vi "TEST_L1_COMPLETE_V2.vi"() -> ()   [LabVIEW 2012]
uses:
  <vilib>/Utility/NIReport.llb/NI_report.lvclass
  <vilib>/Utility/NIReport.llb/HTML/NI_HTML.lvclass
  Sum_Abrilader/L0_Sum_Adder Folder/C/Program Files/National Instruments/LabVIEW 2012/instr.lib/Agilent 8000 Series/Public/Data/Low Level/Fetch Measurement (More).vi
  <instrlib>/Agilent 8000 Series/Agilent 8000 Series.lvlib
  Sum_Abrilader/L0_Sum_Adder Folder/C/Program Files/National Instruments/LabVIEW 2012/instr.lib/Agilent 81150/Agilent 81150.lvlib
panel:
  in  "Default register":u16[](array[numeric])=[2389, 32764, 32767, 32767, 16384, 160, 6656]
  out "Current Channel":i32
  in  "Pulse Amplitudes":dbl[](array[numeric])=[0.3]
  out "IPR_count":u32=1000
  in  "step":i32=10
  in  "min DT":i32
  in  "max DT":dbl=200.0
  in  "Gains":dbl[](array[numeric])=[0.96, 0.97, 0.98, 0.88, 1.0, 1.0, 0.99]
  in  "Instrument VISA in":T1={"AWG VISA"="AgilentGenerator1", "Oscilloscope  VISA "="AgilentOsciloscope", "Integration Board IP"="172.16.17.48", "connection ID"=refnum, "report out"=refnum, "report file path"=path "C:/Users/omartinez/Desktop/L0nL1_Results"}
  out "data out serial":string="empty_read_bufferwrittingempty_read_bufferwritting2"
  in  "Combination\n  (Act High)":i32 min=0 max=127 step=1 format="%b"
  in  "Single/Comb":bool=TRUE
  in  "Single Channel Enable":i32(slide) scale=0.0..6.0
  out "error out":errorcluster
  in  "error in":errorcluster
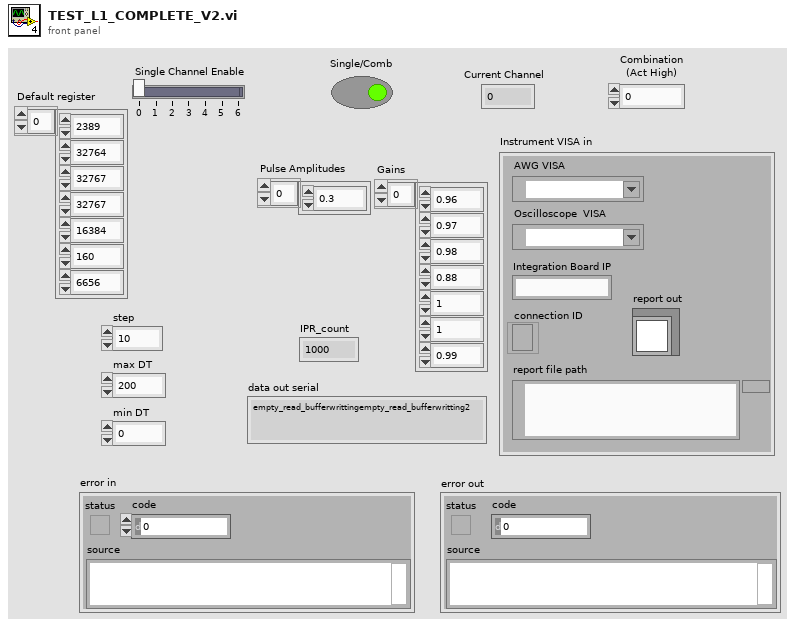
[diagram p1: front panel]
types:
  T1 = cluster{"AWG VISA":refnum<visa-resource-name>, "Oscilloscope  VISA ":refnum<visa-resource-name>, "Integration Board IP":string, "connection ID":refnum<k5>, "report out":refnum<class "NI_report.lvclass">, "report file path":path}
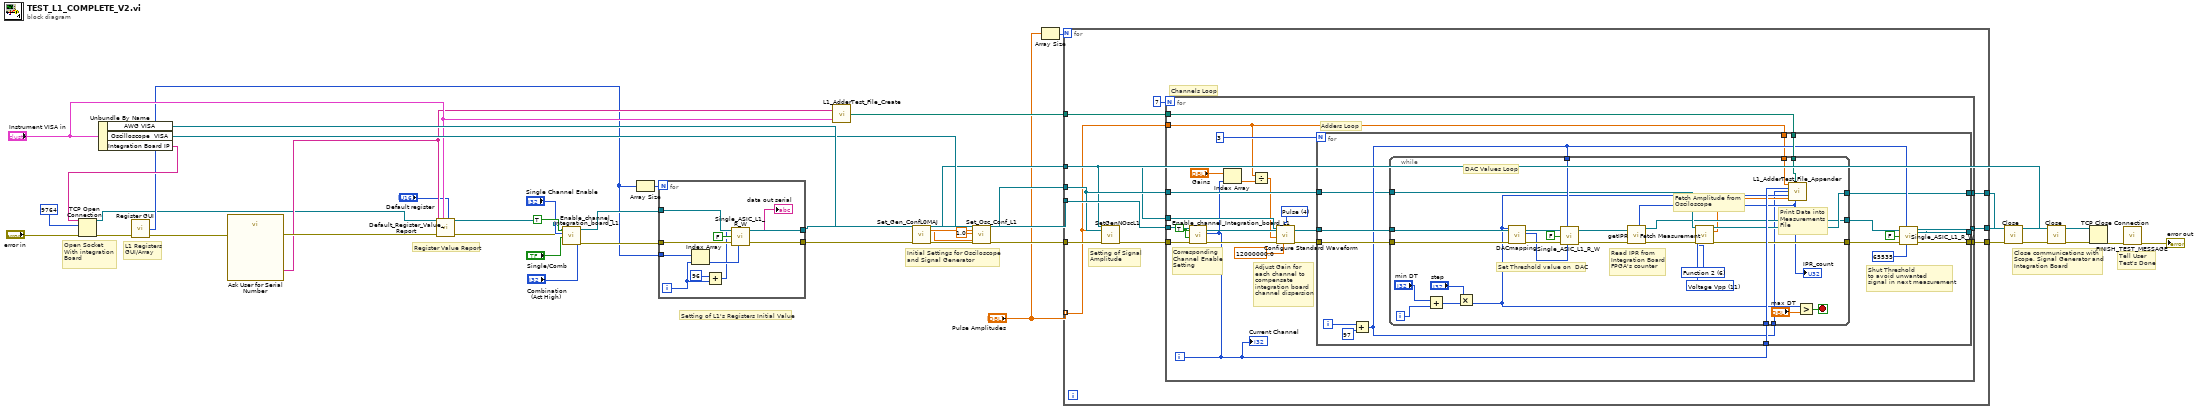
[diagram p0: block diagram]
diagram:
  # "Register Value Report"
  # "Tell User\nTest's Done"
  # "Close communications with \nScope, Signal Generator and \nIntegration Board"
  # "Initial Settings for Osciloscope\nand Signal Generator"
  # "Setting of L1's Registers Initial Value"
  # "L1 Registers\nGUI/Array"
  # "Open Socket\nWith integration \nBoard"
  n1 = Unbundle By Name("Instrument VISA in") -> ("AWG VISA"=w25:refnum<visa-resource-name>, "Oscilloscope  VISA"=w24:refnum<visa-resource-name>, "Integration Board IP"=w31:string)
  n2 = TCP Open Connection(address=w31, remote port or service name=9764, error in (no error)="error in") -> (connection ID=w3:refnum<k5>, error out=w12:errorcluster)  [unwired: 2 in]
  n3 = call "Register GUI.vi"("error in (no error)"=w12) -> ("error out"=w11:errorcluster, "REG ARRAy"=w4:u32[])  [unwired: 3 in]
  n4 = call "Ask User for Serial Number"("error in (no error)"=w11) -> ("Serial Number"=w5:string, "error out"=w7:errorcluster)  [unwired: 16 in, 1 out]
  n5 = call "Default_Register_Value_Report.vi"("Default register"="Default register", "input cluster"="Instrument VISA in", "error out"=w7, "Serial Number"=w5, "connection ID"=w3) -> ("error out 2"=w8:errorcluster, "connection ID out"=w2:refnum<k5>)  [unwired: 4 in, 1 out]
  n6 = call "Enable_channel_Integration_board_L1.vi"("Cobination"="Combination\n  (Act High)", "Enable  L1 single  Input"="Single Channel Enable", "error in (no error)"=w8, "SingleIN/#Combination"="Single/Comb", "#Enable all L1"=TRUE, "connection ID"=w2) -> ("error out"=w9:errorcluster, "connection ID out"=w33:refnum<k5>)
  n7 = Array Size(array=w4) -> (size(s)=w34:i32)
  n8 = for {
    N: w34 -> [_]
    tunnel: w9 -> [w52]
    tunnel: w4 -> [w51]
    tunnel: w33 -> [w50]
    tunnel: [w49] -> w29
    tunnel: [w48] -> w10
    i -> [w43]
    n9 = Index Array(array=w51, index=w43) -> (element=w47:u32)
    n10 = Add(x=96 ("y"), y=w43) -> (x+y=w45:i32)
    n11 = call "Single_ASIC_L1_R_W.vi"("connection ID"=w50, "Register or channel"=w45, "RD/#WR"=FALSE, "error in (no error)"=w52, "Data"=w47) -> ("data out serial"=→"data out serial":string, "connection ID out"=w49:refnum<k5>, "error out"=w48:errorcluster)  [unwired: 1 in, 1 out]
  }
  n12 = call "L1_AdderTest_File_Create.vi"("input cluster"="Instrument VISA in", "Serial Number"=w5) -> ("appended path"=w30:path)
  n13 = call "Set_Gen_ConfL0MAJ.vi"("AWG VISA"=w25, "error in (no error)"=w10) -> ("Amplitude 1 OUT"=w27:dbl, "VISA resource name out"=w16:refnum<visa-resource-name>, "Pulse Width in seconds 1 OUT"=w26:dbl, "error out"=w28:errorcluster)  [unwired: 10 in, 4 out]
  n14 = call "Set_Osc_Conf_L1.vi"("VISA resource name"=w24, "Amplitude IN"=w27, "Trigger Level IN"=1.0, "Pulse Width in seconds IN"=w26, "error in (no error)"=w28) -> ("VISA resource name out"=w18:refnum<visa-resource-name>, "error out"=w19:errorcluster)  [unwired: 13 in]
  n15 = Array Size(array="Pulse Amplitudes") -> (size(s)=w14:i32)
  n16 = for {
    N: w14 -> [_]
    tunnel: [w63] -> w32
    tunnel: w30 -> [w61]
    tunnel: w29 -> [w60]
    tunnel: [w59] -> w23
    tunnel: [w58] -> w20
    tunnel: w19 -> [w57]
    tunnel: w18 -> [w55]
    tunnel: w16 -> [w54]
    tunnel: "Pulse Amplitudes" -> [w53] mode=indexing
    # "Setting of Signal\nAmplitude"
    # "Channels Loop"
    n17 = call "SetGenNOscL1.vi"("Input Voltage"=w53, "error in (no error)"=w57, "VISA resource name"=w55, "AWG VISA"=w54) -> ("error out 2"=w56:errorcluster)  [unwired: 7 in]
    n18 = for {
      N: 7 -> [_]
      tunnel: [w83] -> w59
      tunnel: [w81] -> w63
      tunnel: w60 -> [w79]
      tunnel: w61 -> [w77]
      tunnel: w53 -> [w68]
      tunnel: w56 -> [w76]
      tunnel: w55 -> [w75]
      tunnel: [w74] -> w58
      tunnel: w54 -> [w70]
      i -> [w69]
      w73 = u16 4 items=["Sine", "Square", "Ramp Up", "Ramp Down", "Pulse", "Noise", "DC"] ("Waveform (0: Sine)")
      w78 = TRUE ("#Enable all L1")
      # "Adjust Gain for\neach channel to\ncompensate \nintegration board\nchannel dispersion"
      # "Corresponding\nChannel Enable\nSetting"
      # "Adders Loop"
      n19 = call "Enable_channel_Integration_board_L1.vi"("Enable  L1 single  Input"=w69, "error in (no error)"=w76, "SingleIN/#Combination"=w78, "#Enable all L1"=w78, "connection ID"=w79) -> ("error out"=w72:errorcluster, "connection ID out"=w80:refnum<k5>)  [unwired: 1 in]
      n20 = Index Array(array="Gains", index=w69) -> (element=w64:dbl)
      n21 = Divide(x=w68, y=w64) -> (x/y=w67:dbl)
      n22 = call <instrlib>:"Configure Standard Waveform.vi"("Frequency (1000.0 Hz)"=12000000.0, "Waveform (0: Sine)"=w73, "error in (no error)"=w72, "Amplitude (1.0 Vpp)"=w67, "VISA resource name"=w70) -> ("error out"=w71:errorcluster)  [unwired: 5 in, 1 out]
      n23 = for {
        N: 3 -> [_]
        tunnel: w80 -> [w99]
        tunnel: w71 -> [w96]
        tunnel: [w95] -> w83
        tunnel: [w93] -> w81
        tunnel: w77 -> [w90]
        tunnel: w69 -> [w89]
        tunnel: w68 -> [w87]
        tunnel: w75 -> [w85]
        tunnel: [w84] -> w74
        i -> [w97]
        # "Shut Threshold\nto avoid unwanted\nsignal in next measurement"
        n24 = Add(x=w97, y=97) -> (x+y=w88:i32)
        n25 = while {
          tunnel: w99 -> [w127]
          tunnel: w88 -> [w125]
          tunnel: w96 -> [w124]
          tunnel: [w109] -> w94
          tunnel: [w115] -> w86
          tunnel: w90 -> [w120]
          tunnel: w89 -> [w119]
          tunnel: w88 -> [w100]
          tunnel: w87 -> [w118]
          tunnel: w85 -> [w114]
          tunnel: [w113] -> w84
          i -> [w103]
          stop <- w121 stop-if-true
          w117 = 11 items=["Rise Time", "Fall Time", "Frequency", "Period", "Voltage RMS(AC)", "Voltage RMS(DC)", "Voltage RMS (AC,cycle)", "Voltage RMS (DC,cycle)", "Voltage Max", "Voltage Min", "Voltage Middle", "Voltage Vpp", "Voltage High", "Voltage Low", "Voltage Average", "Voltage Average (cycle)", "Width Negative", "Width Positive", "Duty Cycle Positive", "Amplitude", "Overshoot", "Preshoot", "Voltage Base", "Voltage Upper", "Time Max", "Time Min", "Color Grade Crossing", "Color Grade Eye Width", "Color Grade Eye Height", "Color Grade Eye Q-Factory", "Color Grade Eye Duty Cycle Distortion(Percent)", "Color Grade Eye Duty Cycle Distortion(Time)", "Color Grade Eye Jitter(PP)", "Color Grade Eye Width(RMS)", "Cycle-cycle Duty Jitter(Rising)", "Cycle-cycle Duty Jitter(Falling)", "Cycle-cycle Jitter(Rising)", "Cycle-cycle Jitter(Falling)", "Cycle-cycle - Width", "Cycle-cycle + Width", "Date Rate", "Unit Interval", "FFT Delta Frequency", "FFT Delta Magnitude", "FFT Frequency", "FFT Magnitude", "Slew Rate", "Area (Entire Display)", "Area(Single Cycle)", "Duty Cycle (Rising)", "Duty Cycle (Falling)"] ("Measurement Function (0: Rise Time)")
          w116 = 6 items=["Channel 1"=1, "Channel 2"=2, "Channel 3"=3, "Channel 4"=4, "Function 1"=5, "Function 2"=6, "Function 3"=7, "Function 4"=8, "Memory 1"=9, "Memory 2"=10, "Memory 3"=11, "Memory 4"=12] ("Channel (1: Channel 1)")
          # "Print Data into\nMeasurements \nFile"
          # "Fetch Amplitude from\nOsciloscope"
          # "Read IPR from \nIntegration Board\nFPGA's counter"
          # "Set Threshold value on  DAC"
          # "DAC Values Loop"
          n26 = Add(x="min DT", y=w103) -> (x+y=w106:i32)
          n27 = Multiply(x="step", y=w106) -> (x*y=w102:i32)
          n28 = call "DACmapping.vi"("error in (no error)"=w124, "DAC_TH2"=w102) -> ("error out"=w123:errorcluster, "COMB DEC"=w122:u32)  [unwired: 8 in]
          n29 = call "Single_ASIC_L1_R_W.vi"("connection ID"=w127, "Register or channel"=w125, "RD/#WR"=FALSE, "error in (no error)"=w123, "Data"=w122) -> ("connection ID out"=w110:refnum<k5>, "error out"=w112:errorcluster)  [unwired: 1 in, 2 out]
          n30 = call "getIPR.vi"("error in"=w112, "connection ID"=w110) -> ("error out"=w111:errorcluster, "connection ID out"=w109:refnum<k5>, "IPR_count"=w108:u32)  [unwired: 6 in, 1 out]
          "IPR_count" <- w108
          n31 = call-poly "Fetch Measurement.vi"("VISA resource name"=w114, "Channel (1: Channel 1)"=w116, "Measurement Function (0: Rise Time)"=w117, "error in (no error)"=w111) -> ("VISA resource name out"=w113:refnum<visa-resource-name>, "Measurement"=w107:dbl, "error out"=w115:errorcluster)  [unwired: 9 in]
          n32 = call "L1_AdderTest_File_Appender.vi"("Vin"=w118, "file path (dialog if empty)"=w120, "CH"=w119, "Active Adder"=w100, "DAC Level"=w102, "Vmeas"=w107, "IPR"=w108) -> ()  [unwired: 9 in]
          n33 = Greater?(x=w102, y="max DT") -> (0:w121:bool)
        }
        n34 = call "Single_ASIC_L1_R_W.vi"("connection ID"=w94, "Register or channel"=w88, "RD/#WR"=FALSE, "error in (no error)"=w86, "Data"=u32 65535 ("COMB DEC")) -> ("connection ID out"=w93:refnum<k5>, "error out"=w95:errorcluster)  [unwired: 1 in, 2 out]
      }
      "Current Channel" <- w69
    }
  }
  n35 = call <instrlib>:"Close.vi"("error in (no error)"=w23, "VISA resource name"=w20) -> ("error out"=w22:errorcluster)  [unwired: 9 in]
  n36 = call <instrlib>:"Close.vi"("error in (no error)"=w22, "VISA resource name"=w16) -> ("error out"=w21:errorcluster)  [unwired: 9 in]
  n37 = TCP Close Connection(connection ID=w32, error in (no error)=w21) -> (error out=w39:errorcluster)  [unwired: 1 in, 1 out]
  n38 = call "FINISH_TEST_MESSAGE.vi"("error in"=w39) -> ("error out"=→"error out":errorcluster)  [unwired: 10 in]
